vi "Get latest folder based on date mod.vi"(8 "error in":errorcluster, 11 "path":path=path "C:/perforce") -> (0 "error out":errorcluster, 3 "appended path":path)   [LabVIEW 2013]
panel:
  out "max index(es)":i32
  out "max value":timestamp
  out "folder names":string[](array[string])
  out "Array":timestamp[](array[timestamp])
  out "directory":bool
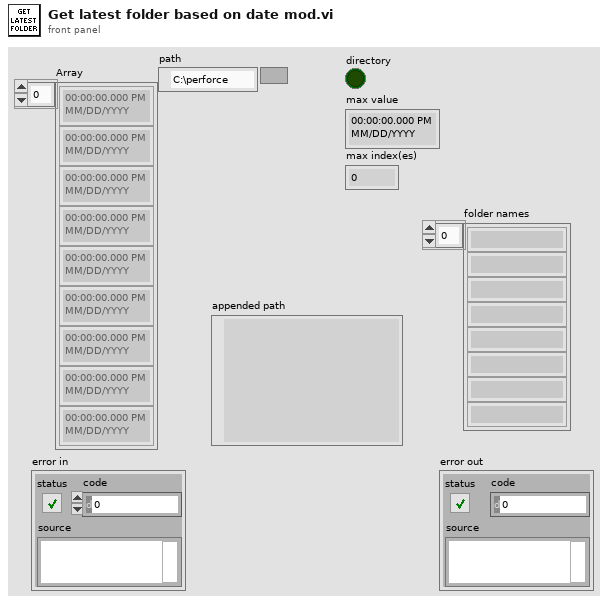
[diagram p1: front panel]
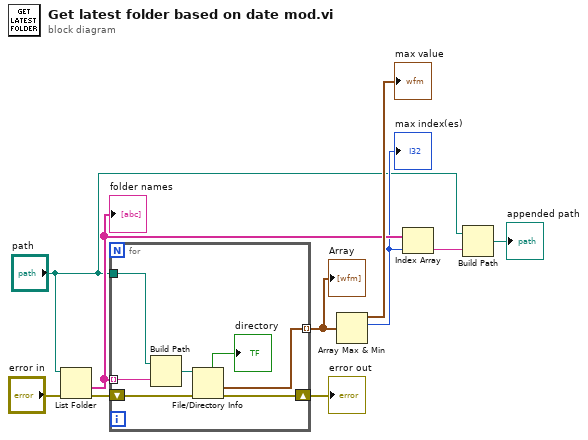
[diagram p0: block diagram]
diagram:
  n1 = List Folder(path="path", error in="error in") -> (folder names=w8:string[], error out=w2:errorcluster)  [unwired: 2 in, 2 out]
  "folder names" <- w8
  n2 = for {
    tunnel: "path" -> [w15]
    tunnel: [w16] -> w10 mode=indexing
    tunnel: w8 -> [w14] mode=indexing
    shift-right: [w12] -> w1
    shift-left: w2 -> [w11]
    n3 = Build Path(base path=w15, name or relative path=w14) -> (appended path=w13:path)
    n4 = File/Directory Info(path=w13, error in=w11) -> (directory=→"directory":bool, last mod=w16:timestamp, error out=w12:errorcluster)  [unwired: 4 out]
  }
  "Array" <- w10
  "error out" <- w1
  n5 = Array Max & Min(array=w10) -> (max value=→"max value":timestamp, max index (indices)=w7:i32)  [unwired: 2 out]
  "max index(es)" <- w7
  n6 = Index Array(array=w8, index=w7) -> (element=w6:string)
  n7 = Build Path(base path="path", name or relative path=w6) -> (appended path=→"appended path":path)
